vi "STM Connection Manager.vi"(6 "Properties In":T1, 8 "error in (no error)":errorcluster, 9 "Method":T2, 10 "Index":i32, 11 "Connection In":refnum<k5>) -> (0 "error out":errorcluster, 1 "Number of \nConnections":i32, 2 "All Connections":refnum<k5>[](array[refnum]), 3 "Connection Out":refnum<k5>, 4 "Properties out":T1, 5 "All Properties":T1[](array[typedef]))   [LabVIEW 2014, in "QwaveSys Raspberry Pi Library.lvlib"]
doc: "This VI maintains the list of host connections."
uses:
  _SubVIs/TypeDefs/stm_ConnectionMethod.ctl
  _SubVIs/TypeDefs/stm_ConnectionProperties.ctl
  QwaveSys Raspberry Pi Library.lvlib
panel:
  out "Number of properties":i32
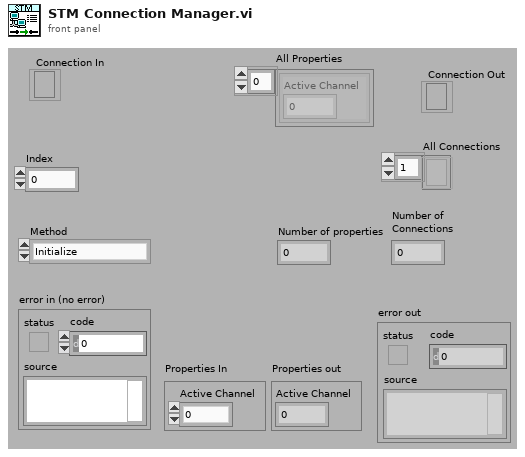
[diagram p1: front panel]
types:
  T1 = typedef "QwaveSys Raspberry Pi Library.lvlib/stm_ConnectionProperties.ctl" = cluster{"Active Channel":i32}
  T2 = typedef "QwaveSys Raspberry Pi Library.lvlib/stm_ConnectionMethod.ctl" = enum16{"Initialize", "Add Connection", "Set Properties", "Get Connection(s)", "Close Connection", "Close Connections"}
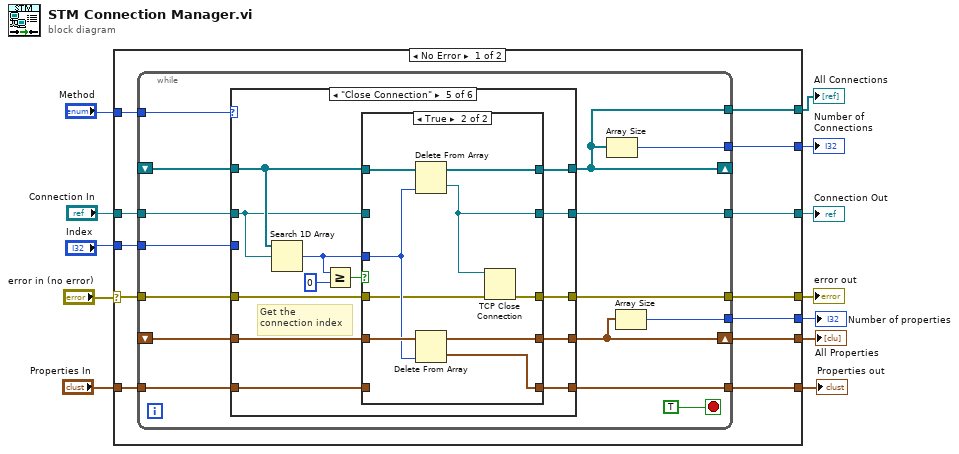
[diagram p0: block diagram]
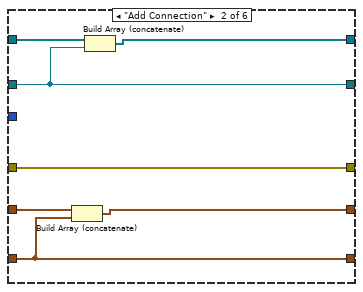
[diagram p3: hidden frame]
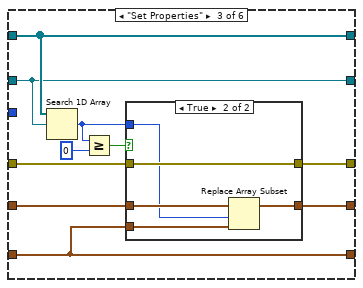
[diagram p4: hidden frame]
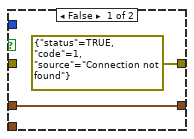
[diagram p5: hidden frame]
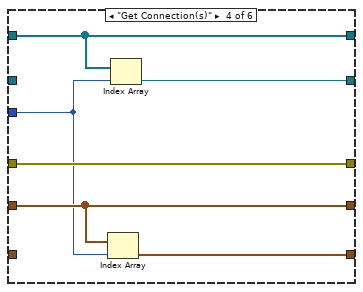
[diagram p6: hidden frame]
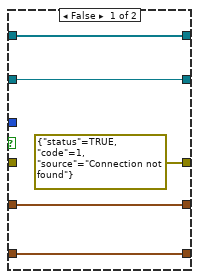
[diagram p7: hidden frame]
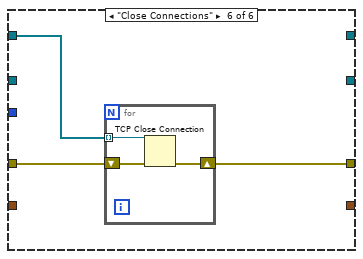
[diagram p8: hidden frame]
diagram:
  n1 = case shown="No Error" "error in (no error)" {
    selector: "error in (no error)" -> [w24 w105]
    tunnel: [w23 w105] -> w11
    tunnel: "Index" -> [w22 _]
    tunnel: "Method" -> [w21 _]
    tunnel: "Connection In" -> [w20 w104]
    tunnel: [w19 _] -> w7
    tunnel: [w18 _] -> w6
    tunnel: [w17 w104] -> w5
    tunnel: "Properties In" -> [w16 _]
    tunnel: [w15 _] -> w3
    tunnel: [w14 _] -> w2
    tunnel: [w13 _] -> w1
    frame No Error {
      n2 = while {
        shift-right: [w31] -> _
        shift-left: _ -> [w38]
        tunnel: w24 -> [w37]
        tunnel: [w36] -> w23
        tunnel: w22 -> [w35]
        tunnel: w21 -> [w34]
        tunnel: w20 -> [w33]
        tunnel: [w32] -> w19
        tunnel: [w31] -> w18
        tunnel: [w30] -> w17
        shift-right: [w27] -> w14
        shift-left: _ -> [w29]
        tunnel: w16 -> [w28]
        tunnel: [w26] -> w15
        tunnel: [w25] -> w13
        stop <- TRUE stop-if-true
        n3 = case shown="\"Close Connection\"" w34 {
          tunnel: w38 -> [_ w47 w56 w70 w83 w100]
          tunnel: w33 -> [_ w45 w55 _ w75 _]
          tunnel: [_ w46 w56 w70 w79 _] -> w31
          tunnel: [_ w45 w55 w69 w78 _] -> w30
          tunnel: [w40 w44 w52 w68 w77 w98] -> w36
          tunnel: w37 -> [w40 w44 w53 w68 w76 w99]
          tunnel: w35 -> [_ _ _ w66 _ _]
          tunnel: w29 -> [_ w43 w51 w67 w74 _]
          tunnel: w28 -> [_ w41 w48 _ w71 _]
          tunnel: [_ w42 w49 w67 w73 _] -> w27
          tunnel: [_ w41 w48 w65 w72 _] -> w25
          frame "Initialize" {
          }
          frame "Add Connection" {
            n4 = Build Array (concatenate)(w43, w41) -> (w42:T1[])
            n5 = Build Array (concatenate)(w47, w45) -> (w46:refnum<k5>[])
          }
          frame "Set Properties" {
            n6 = Search 1D Array(1D array=w56, element=w55) -> (index of element=w50:i32)  [unwired: 1 out]
            n7 = Greater Or Equal?(x=w50, y=0) -> (x >= y?=w54:bool)
            n8 = case shown="True" w54 {
              tunnel: w53 -> [_ w64]
              tunnel: [errorcluster {"status"=TRUE, "code"=1, "source"="Connection not found"} ("error out 2") w64] -> w52
              tunnel: w51 -> [w59 w63]
              tunnel: w50 -> [_ w62]
              tunnel: w48 -> [_ w61]
              tunnel: [w59 w60] -> w49
              frame False {
              }
              frame True {
                n9 = Replace Array Subset(array=w63, new element=w61, index=w62) -> (w60:T1[])
              }
            }
          }
          frame "Get Connection(s)" {
            n10 = Index Array(array=w67, index=w66) -> (element=w65:T1)
            n11 = Index Array(array=w70, index=w66) -> (element=w69:refnum<k5>)
          }
          frame "Close Connection" {
            # "Get the \nconnection index"
            n12 = Search 1D Array(1D array=w83, element=w75) -> (index of element=w82:i32)  [unwired: 1 out]
            n13 = Greater Or Equal?(x=w82, y=0) -> (x >= y?=w80:bool)
            n14 = case shown="True" w80 {
              tunnel: w83 -> [w88 w96]
              tunnel: w82 -> [_ w93]
              tunnel: [w88 w97] -> w79
              tunnel: [w86 w89] -> w78
              tunnel: [errorcluster {"status"=TRUE, "code"=1, "source"="Connection not found"} ("error out 2") w91] -> w77
              tunnel: w76 -> [_ w90]
              tunnel: w75 -> [w86 _]
              tunnel: w74 -> [w85 w95]
              tunnel: [w85 w94] -> w73
              tunnel: [w84 w92] -> w72
              tunnel: w71 -> [w84 _]
              frame False {
              }
              frame True {
                n15 = Delete From Array(array=w96, index=w93) -> (deleted portion=w89:refnum<k5>, array with subset deleted=w97:refnum<k5>[])  [unwired: 1 in]
                n16 = Delete From Array(array=w95, index=w93) -> (deleted portion=w92:T1, array with subset deleted=w94:T1[])  [unwired: 1 in]
                n17 = TCP Close Connection(connection ID=w89, error in (no error)=w90) -> (error out=w91:errorcluster)  [unwired: 2 out]
              }
            }
          }
          frame "Close Connections" {
            n18 = for {
              tunnel: w100 -> [w103] mode=indexing
              shift-right: [w101] -> w98
              shift-left: w99 -> [w102]
              n19 = TCP Close Connection(connection ID=w103, error in (no error)=w102) -> (error out=w101:errorcluster)  [unwired: 2 out]
            }
          }
        }
        n20 = Array Size(array=w31) -> (size(s)=w32:i32)
        n21 = Array Size(array=w27) -> (size(s)=w26:i32)
      }
    }
    frame Error {
    }
  }
  "error out" <- w11
  "Number of \nConnections" <- w7
  "All Connections" <- w6
  "Connection Out" <- w5
  "All Properties" <- w2
  "Properties out" <- w1
  "Number of properties" <- w3
